vi "RunVIPath.vi"(8 "Error In":errorcluster, 9 "Settings":T1, 10 "JSON Input":string, 11 "VI Path":path) -> (0 "Error Out":errorcluster, 2 "JSON Output":string)   [LabVIEW 2019, in "LabJSON.lvlib"]
doc: "Take JSON as input, run the VI, and return the output as JSON"
uses:
  LabJSON.lvlib
  Typedefs/Settings.ctl
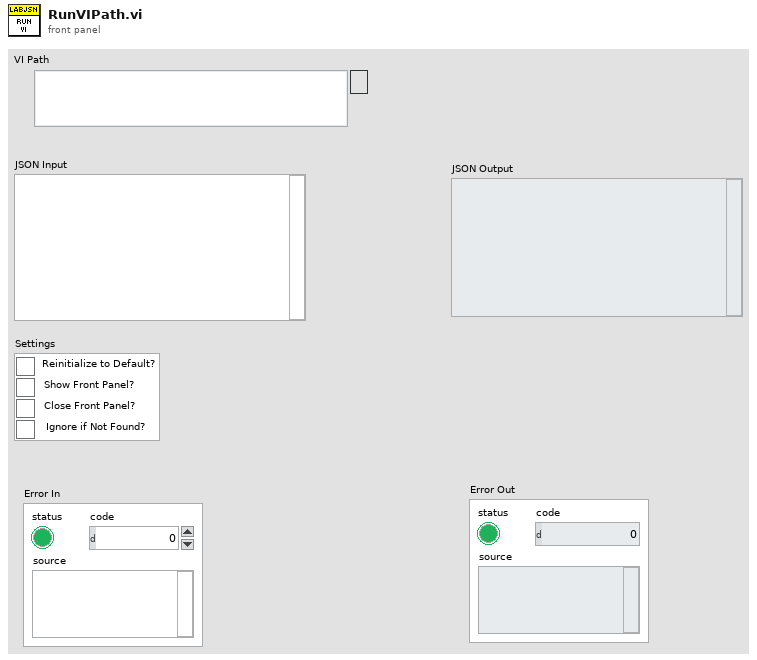
[diagram p1: front panel]
types:
  T1 = typedef "LabJSON.lvlib/Settings.ctl" = cluster{"Reinitialize to Default?":bool, "Show Front Panel?":bool, "Close Front Panel?":bool, "Ignore if Not Found?":bool}
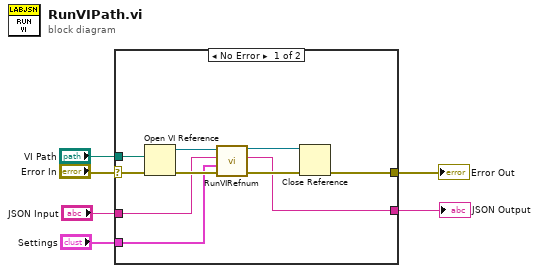
[diagram p0: block diagram]
diagram:
  n1 = case shown="No Error" "Error In" {
    selector: "Error In" -> [w16 w17]
    tunnel: "VI Path" -> [w15 _]
    tunnel: "JSON Input" -> [w12 _]
    tunnel: [w9 w17] -> w3
    tunnel: [w8 _] -> w2
    tunnel: "Settings" -> [w7 _]
    frame No Error {
      n2 = Open VI Reference(vi path=w15, error in (no error)=w16) -> (vi reference=w13:refnum<vi>, error out=w14:errorcluster)  [unwired: 4 in]
      n3 = call "RunVIRefnum.vi"("Error In"=w14, "Settings"=w7, "JSON Input"=w12, "VI Refnum In"=w13) -> ("Error Out"=w11:errorcluster, "JSON Output"=w8:string, "VI Refnum Out"=w10:refnum<vi>)  [unwired: 5 in]
      n4 = Close Reference(reference=w10, error in (no error)=w11) -> (error out=w9:errorcluster)
    }
    frame Error {
    }
  }
  "JSON Output" <- w2
  "Error Out" <- w3
